vi "Initialize.vi"(8 "error in":errorcluster) -> (0 "error out":errorcluster, 3 "CoreOOB_Rx out":refnum<class "CIFCoreOOB_Rx.lvclass">)   [LabVIEW 2021, in "CIFCoreOOB_Rx.lvclass"]
uses:
  CIFCoreOOB_Rx.lvclass
  D:/dev/CIF-LVCore/src/CIFUtilities/CIFOutOfBand/CIFOutOfBand.lvclass
  Typedef/Channel Connection Data.ctl
  CIFCoreOOB_Rx.lvclass/CIFCoreOOB_Rx.ctl
  Common/Typedef/Common Plugin Configuration.ctl
  Typedef/Template Payload.ctl
  CIFUtilities/CIFOutOfBand/CIFOutOfBand.lvclass/CIFOutOfBand.ctl
  CIFUtilities/CIFOutOfBand/CIFOutOfBand.lvclass
  Common/CIFCoreCommon.lvlib
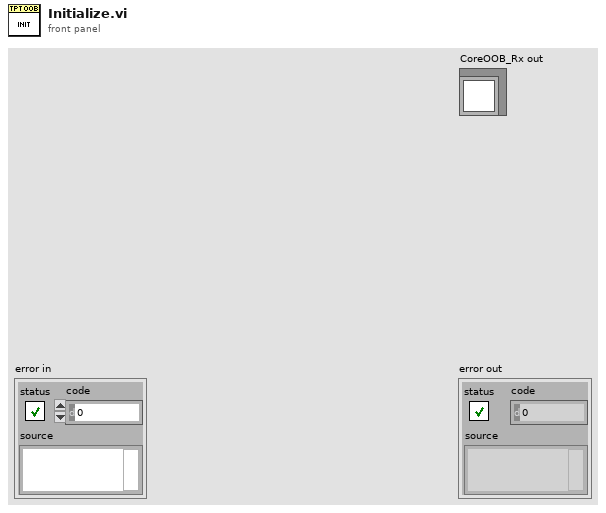
[diagram p1: front panel]
types:
  T1 = typedef "CIFCoreOOB_Rx.lvclass/Channel Connection Data.ctl" = cluster{"Publisher Name":string, "Subscriber Name":string, "Connection Data":u8[]}
  T2 = typedef "CIFCoreOOB_Rx.lvclass/Template Payload.ctl" = cluster{"Config Data":variant, "Connections":T1[]}
  T3 = typedef "CIFCoreCommon.lvlib/Common Plugin Configuration.ctl" = cluster{"Period (s)":dbl, "Offset (us)":i32, "ClockID":u8, "Priority":i32, "Processor":i32}
  T4 = typedef "CIFCoreOOB_Rx.lvclass/Command Setting Control.ctl" = cluster{"Enum":T5, "U8":u8, " Payload":bool}
  T5 = typedef "CIFCoreOOB_Rx.lvclass/OOB Core Commands.ctl" = enum8{"Start", "Pause", "Stop", "RefreshStats", "UpdateConfig", "Connect Channel"}
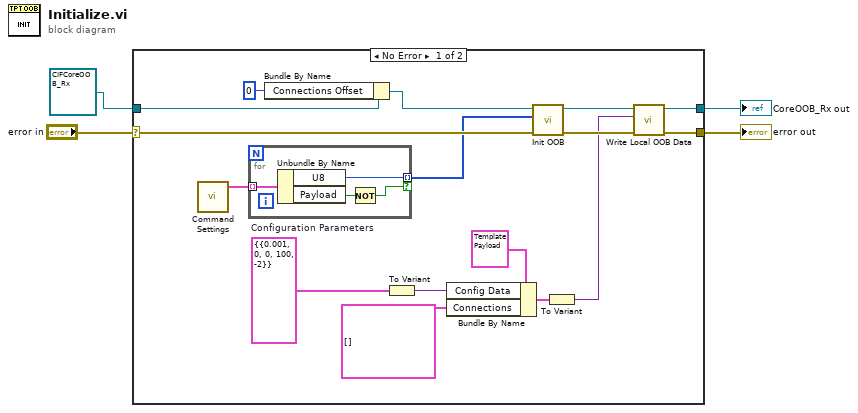
[diagram p0: block diagram]
diagram:
  n1 = case shown="No Error" "error in" {
    selector: "error in" -> [w20 w26]
    tunnel: [w14 w26] -> w3
    tunnel: [w15 w25] -> w2
    tunnel: refnum<class "CIFCoreOOB_Rx.lvclass"> refnum ("CifLvTemplateOutOfBand in") -> [w8 w25]
    frame No Error {
      w10 = cluster{"Common":T3} {"Common"={"Period (s)"=0.001, "Offset (us)"=0, "ClockID"=0, "Priority"=100, "Processor"=-2}}  # Configuration Parameters
      n2 = call "Command Settings.vi"() -> ("Command Settings"=w19:T4[])  [unwired: 5 in]
      n3 = for {
        tunnel: w19 -> [w24] mode=indexing
        tunnel: [w23] -> w18 mode=indexing if=w21
        n4 = Unbundle By Name(w24) -> ("U8"=w23:u8, "Payload"=w22:bool)
        n5 = Not(x=w22) -> (.not. x?=w21:bool)
      }
      n6 = Bundle By Name(cluster=w8, "Connections Offset"=0) -> (w6:refnum<class "CIFCoreOOB_Rx.lvclass">)
      n7 = To Variant(anything=w10) -> (Variant=w9:variant)
      n8 = Bundle By Name(cluster=T2 {"Config Data"=variant, "Connections"=[]} ("Template Payload"), "Config Data"=w9, "Connections"=T1[] []) -> (w12:T2)
      n9 = call "Init OOB.vi"("error in (no error)"=w20, "Cases to Skip Payload"=w18, "OOB in"=w6) -> ("error out"=w17:errorcluster, "OOB out"=w16:refnum<class "CIFCoreOOB_Rx.lvclass">)  [unwired: 7 in]
      n10 = To Variant(anything=w12) -> (Variant=w11:variant)
      n11 = call "Write Local OOB Data.vi"("error in"=w17, "Local OOB Data"=w11, "OOB in"=w16) -> ("error out"=w14:errorcluster, "OOB out"=w15:refnum<class "CIFCoreOOB_Rx.lvclass">)  [unwired: 7 in]
    }
    frame Error {
    }
  }
  "error out" <- w3
  "CoreOOB_Rx out" <- w2
